vi "Update UI.vi"(8 "error in (no error)":errorcluster, 10 "String Data":string, 11 "Calling Actor In":refnum<class "Calling Actor.lvclass">) -> (0 "error out":errorcluster, 3 "Calling Actor Out":refnum<class "Calling Actor.lvclass">)   [LabVIEW 2015, in "Calling Actor.lvlib" / "Calling Actor.lvclass"]
uses:
  Calling Actor.lvclass
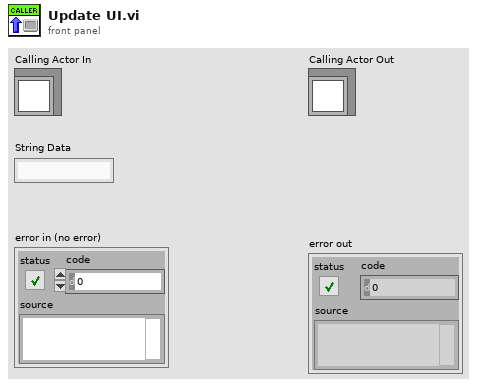
[diagram p1: front panel]
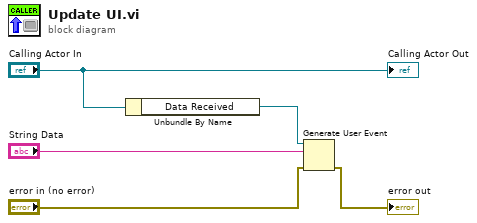
[diagram p0: block diagram]
diagram:
  n1 = Unbundle By Name("Calling Actor In") -> ("Data Received"=w4:refnum<user-event>)
  n2 = Generate User Event(user event=w4, event data cluster="String Data", error in="error in (no error)") -> (error out=→"error out":errorcluster)  [unwired: 1 in, 1 out]
  "Calling Actor Out" <- "Calling Actor In"
